vi "FFT_DAS_GUI.vi"() -> ()   [LabVIEW 2018]
doc: "<b>LITVC - ?????????????????????</b>\n\nMeasures, graphs and logs the data from the LITVC cRIO Chassis. Samples 12 analog channels of raw at kilohertz speeds, and controls starting of test data runs, with triggered control of the appropriate solenoid valves . \n\nSystem scaling and other constants are loaded from the \"LITVC_CFG.TXT\" text file at startup. (The order of the lines must remain the same. ) The Operator must supply a data file path and name at startup. This defaults on the cRIO Controller to: \"C:\\Data\". The software then starts data acquisition and logging, as indicated by the blinking green \"Active\" LED.\n\nPressing \"CAL\" after start will calibrate the system to the cross section of the wire rope.\nTo stop the acquisition, press the Stop button in the upper right. This allows the operator to look at the graphs, error indicators, etc on the status tab.\nTo Exit, press the EXIT button on the Status tab.\n\nVersion 1.0.0:\n 1. Initial version\n\n2010_09_30 Michael Ashe\nmichael.ashe@aztera.com\nmichael.ashe@imaginatics.net\n(860) 961-0876 (Cell)"
uses:
  Common/Controls/GUI_Buttons_23x22_W2K.llb/MacroPlay.ctl
  Common/Controls/GUI_Buttons_23x22_W2K.llb/MacroPause.ctl
  Common/Controls/GUI_Buttons_23x22_W2K.llb/MacroStop.ctl
  Common/Controls/BlockStart Button.ctl
  Common/Controls/BlockEnd Button.ctl
  Common/Controls/FFT_DAS Shift Variables.ctl
  Common/COMM_Queues/Command Queue Cluster.ctl
  Common/WRIS_Config Vars Cluster.ctl
  Common/GUI/Enable Controls API.llb/Action.ctl
  Common/Timing/Controls/StateMachineStates_TEST_TDEF.ctl
  Common/COMM_Queues/Command_Queue_Select.ctl
  Common/StateFile.llb/Actions.ctl
  <vilib>/DAQmx/read.llb/DAQmx Read (Analog 1D DBL NChan 1Samp).vi
  <vilib>/DAQmx/write.llb/DAQmx Write (Analog 1D DBL NChan 1Samp).vi
  <vilib>/DAQmx/read.llb/DAQmx Read (Analog 1D Wfm NChan NSamp).vi
  <vilib>/DAQmx/read.llb/DAQmx Read (Counter DBL 1Chan 1Samp).vi
  Common/Globals/FFT_DAS-Editing Variables_GBL.vi
  <vilib>/DAQmx/miscellaneous.llb/DAQmx Fill In Error Info.vi
  <vilib>/measure/madcrms.llb/Basic Averaged DC-RMS for N Chan.vi
  <vilib>/DAQmx/configure/timing.llb/DAQmx Timing (Sample Clock).vi
  <vilib>/DAQmx/create/channels.llb/DAQmx Create Channel (CI-Frequency).vi
  <vilib>/DAQmx/configure/timing.llb/DAQmx Timing (Implicit).vi
  Common/GUI/Enable Controls.lvlib
  <vilib>/measure/NI_MAPro.lvlib
panel:
  out "SaveAbortedTest":bool
  out "Test Data":dbl[](array[numeric])
  out "Flow":i32
  out "GPM":dbl[](array[numeric])
  out "Hz":dbl[](array[numeric])
  out "DAQWrite":errorcluster
  out "Numeric":i32
  out "StopAllLoops":bool
  out "Flow Meter":bool
  out "Thermocouple":bool
  out "DAQ":bool
  in  "Tab Control":T1(tab)
  out "In Range":bool=TRUE
  in  "Go to Previous Step":bool
  out "Supply Pressure":dbl(knob) scale=0.0..400.0 scale format="%#.1f"
  out "Hz":dbl format="%.1f"
  out "Fuel Temp":dbl(slide) scale=0.0..150.0 scale format="%#.1f"
  out "Flow(GPM)":dbl(knob) scale=0.0..2.0 scale format="%#.1f"
  out "Flow(lbs/hr)":dbl(knob) scale=0.0..1000.0 scale format="%#.1f"
  out "Bypass Pressure (psig)":dbl(knob) scale=0.0..50.0 scale format="%#.1f"
  out "Back Pressure":dbl(knob) scale=0.0..300.0 scale format="%#.1f"
  out "Diff. Pressure":dbl(knob) scale=0.0..60.0 scale format="%#.1f"
  in  "Go to Next Step":bool
  in  "BP Reg Manual":bool
  in  "Control Devices":cluster{"BP Regulator":dbl} {"BP Regulator" scale=0.0..100.0 scale format="%#3.2f%"}
  out "Test Status":T2(ring)
  in  "BlkMrkGrp":cluster{"Block Start":T3, "Block End":T4}
  in  "MacroGroup":T8
  in  "Test Table":string[][](table)=[["", "20", "10", "109 ", "200", " ", " ", " ", " ", " ", " ", " ", " ", " ", " "], ["", "40", "22", "160", "200", "", " ", " ", " ", " ", " ", " ", " ", " ", " "], ["", "10", "32", "400", "500", "", " ", " ", " ", " ", " ", " ", " ", " ", " "]] caption="A/M    Current      Dwell            Min Flow       Max Flow       Actual Flow      Hysteresis"
  out "EditLine":i32=65534
  out "EditCol":i32=65534
  in  "StartTest":bool
  in  "StopTest":bool
  out "ATS Number":string
  out "CalDate":string
  in  "PSID Setpoint":dbl
  in  "Pressure Tolerance":dbl
  out "mA Tolerance":dbl
  out "Parameter Table Out 2":string[][](table) caption="Parameter Table + Comment Out"
  out "BP Output":dbl format="%.2g"
  out "Report Path":path
  out "Template Path":path
  out "Version":string
  in  "Send to Excel":bool
  out "Test Table2":string[][](table)=[["", "20", "10", "109 ", "200", " ", " ", " ", " ", " ", " ", " ", " ", " ", " "], ["", "40", "22", "160", "200", "", " ", " ", " ", " ", " ", " ", " ", " ", " "], ["", "10", "32", "400", "500", "", " ", " ", " ", " ", " ", " ", " ", " ", " "]] caption="Table"
  out "Parameter Table Out":string[][](table)
  out "Flow-Current XY Graph":cluster{cluster{"X":dbl, "Y":dbl}[]}[](graph)
  out "Flow Freq":errorcluster
  out "DAQRead":errorcluster
  out "USB TC 01":errorcluster
  out "TM Config File":path
  out "AI Task":refnum<k21>="AI"
  out "FEM Device":tag="Dev1/ctr0"
  out "Report Path":path
  out "TempCorrection":dbl
  out "Flow Cal":dbl[][](array[numeric])
  out "@Temp Cal Fluid":dbl format="%.1g °F"
  out "SG Cal Fluid":dbl format="%#.6g"
  out "SG Cal Corrected":dbl format="%.3g"
  out "Cal Temp Coe":dbl format="%#.6g"
  out "Current Cal Temp":dbl format="%.1g °F"
  out "Flow lbs/hr":dbl format="%.3g"
  out "Flow(GPM)":dbl format="%#.3g"
  out "SG CAL Corrected":dbl format="%#.3g"
  out "Std H20 Mass @60F":dbl format="%#.3g"
  # "SG CAL Corrected ="
  # "Hz"
  # "GPM"
  # "SG Cal Fluid + Cal Temp Coe*(Temp Cal Fluid-Current Fuel Temp)"
  # "Flow (PPH) ="
  # "Flow(gpm)*60*SG CAL Correct *Standard H20 Mass @60F"
  # "\"Flow Calibration.txt\" is located in the application directory.\n\nMake Changes to that file and relaunch the application\nto initialize the new calibration. \n\n\nIf the file does not exist create one with the exact file\nname above.  Add as many points as needed. Example:\n\nHz, GPM\n0, 0\n2, 100\n10, 1010"
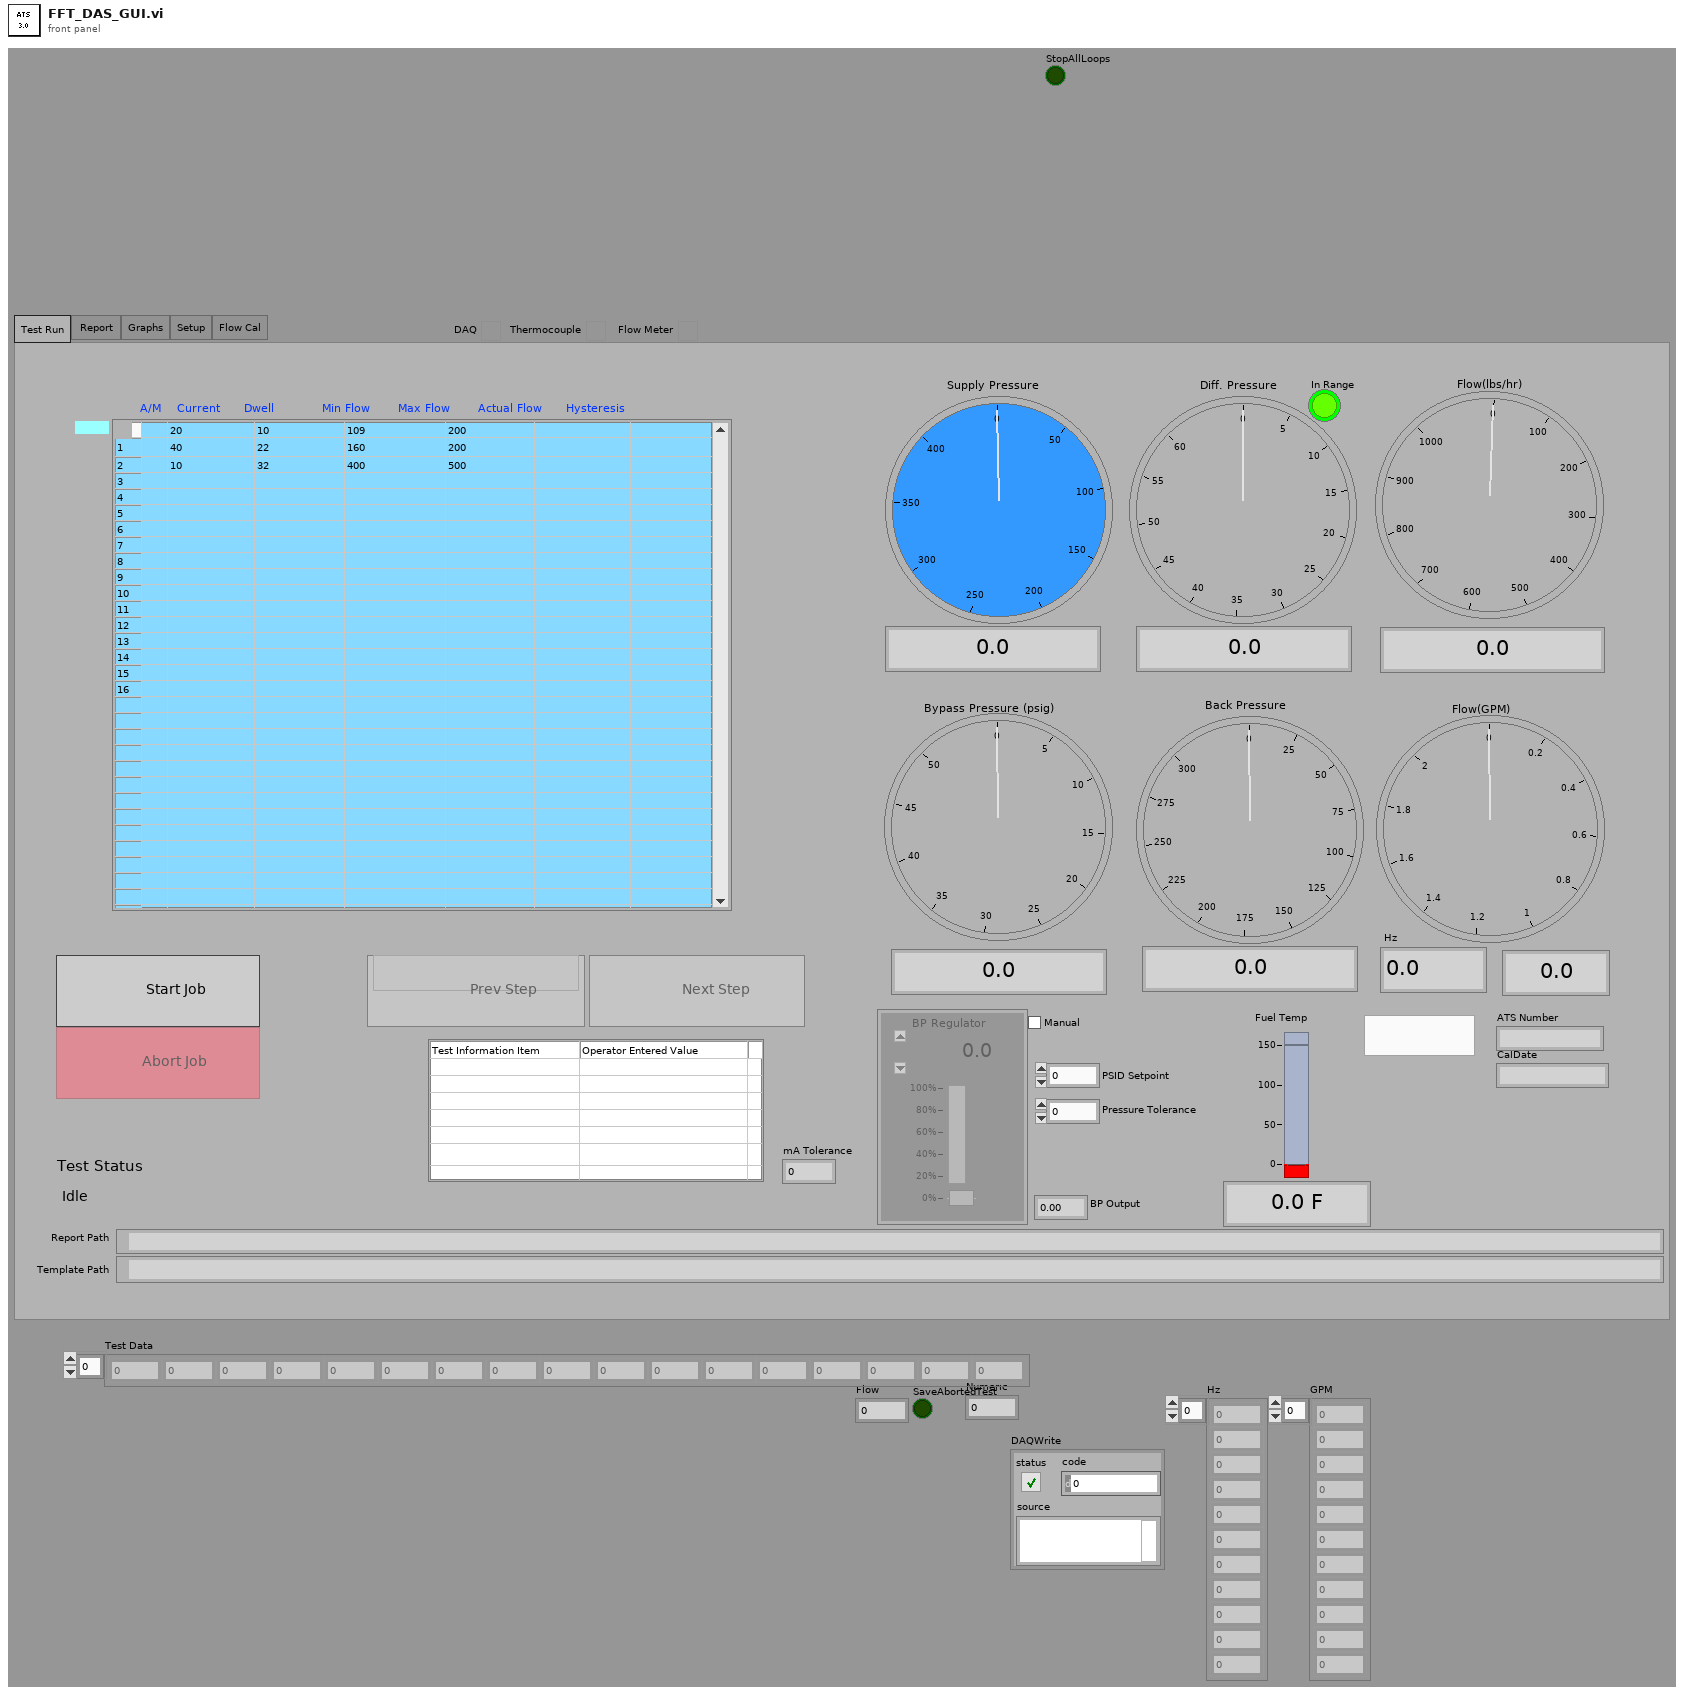
[diagram p1: front panel]
types:
  T1 = enum32{"Test Run", "Report ", "Graphs", "Setup", "Flow Cal"}
  T2 = enum16{"Idle", "Test Running", "Test Paused", "Test Completed"}
  T3 = typedef "BlockStart Button.ctl" = bool
  T4 = typedef "BlockEnd Button.ctl" = bool
  T5 = typedef "MacroPlay.ctl" = bool
  T6 = typedef "MacroPause.ctl" = bool
  T7 = typedef "MacroStop.ctl" = bool
  T8 = cluster{"MacroPlay":T5, "MacroPause":T6, "MacroStop":T7, "MacroName":u16}
  T9 = typedef "FFT_DAS Shift Variables.ctl" = cluster{"queue data":T10, "error":errorcluster, "Q_TO":i32, "WDT_TO":dbl, "LogErrors?":bool, "Main.ini Ref":refnum<k1>, "Connected? 1":bool, "Address 1":string, "Link_Name":string, "Config Vars":T11, "Calibrate":bool, "Cal_Slope-Offset":dbl[][], "TestTable":string[][], "Test Status":enum16{"Idle", "Test Running", "Test Paused", "Test Completed"}, "Parameter Table Out":string[][], "Test Start Time":string, "Test Stop Time":string, "Report Directory":path}
  T10 = typedef "Command Queue Cluster.ctl" = cluster{"Command":string, "Variant Data":variant}
  T11 = typedef "WRIS_Config Vars Cluster.ctl" = cluster{"Distance/Count":dbl, "samples/ch":i32, "Task_TO":dbl, "Kc":dbl, "B":dbl}
  T12 = typedef "Enable Controls.lvlib/Action.ctl" = enum16{"Editor Init", "Init", "Operator Init", "Timed Test Start", "Manual Test Start", "Stop Test", "Close", "Set States"}
  T13 = enum16{"get data", "set data", "Add Data Pair", "initialize"}
  T14 = typedef "StateMachineStates_TEST_TDEF.ctl" = enum16{"Initialize", "Start", "Run Position", "Pause", "Resume", "Get Step", "Force Previous Step", "Force Next Step", "Stay on Current Step"}
  T15 = typedef "Command_Queue_Select.ctl" = enum16{"<no op>", "Destroy Queues", "Send -> State_Machine", "Send -> Client_IO", "Send -> Logging", "Send -> Instrument_IO", "Send -> Tag_Manager", "Send -> Alarms_Shutdowns", "Send -> Control_Loops", "Send -> Server_IO", "Send -> GUI"}
  T16 = typedef "Actions.ctl" = enum16{"Initialize", "Save VI State", "Load VI State", "Delete State", "Get All VI State Names", "Clear All States", "Close Global State File", "Open State File", "Create State File", "Write Data to File", "Exit"}
  T17 = enum8{"Enabled", "Disabled", "Disabled and Grayed Out"}
  T18 = typedef "LVRowAndColumnTypeDef.ctl" = cluster{"Row":i32, "Column":i32}
  T19 = enum16{"STARTUP", "ERROR", "OPEN", "CLOSE", "ENABLE", "DISABLE", "SHUTDOWN"}
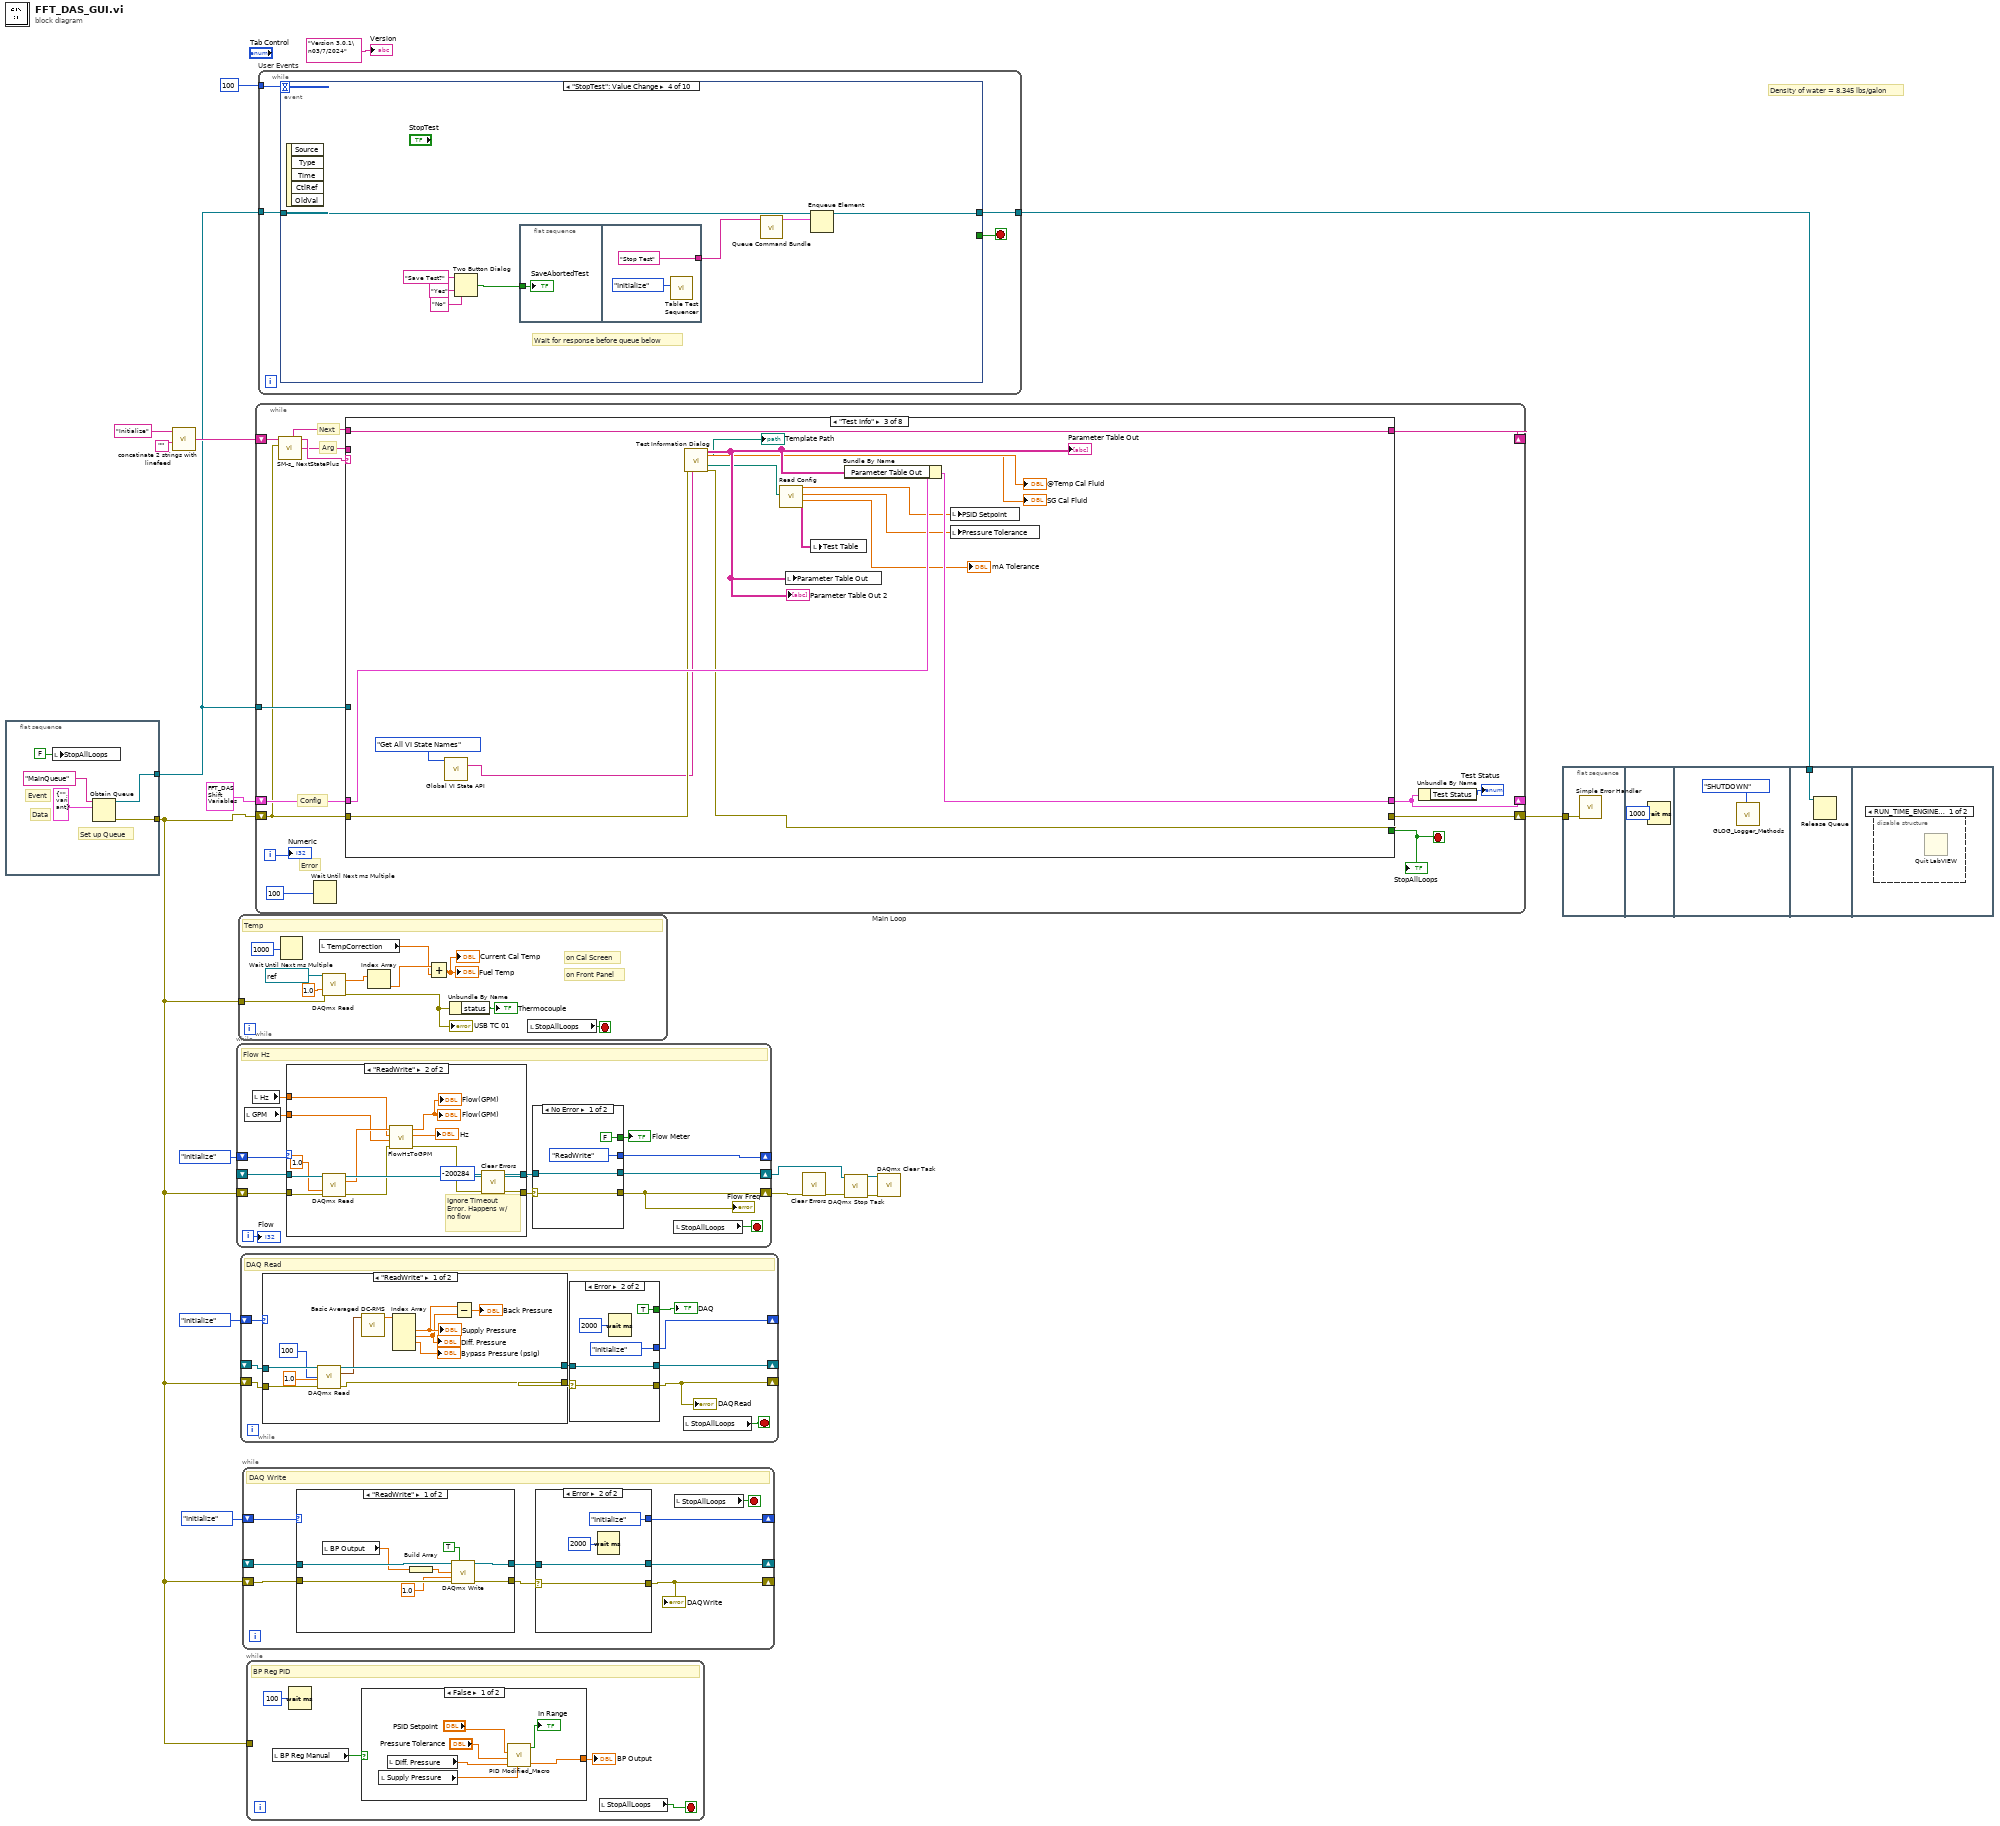
[diagram p0: block diagram]
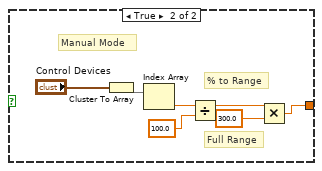
[diagram p2: hidden frame]
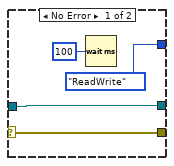
[diagram p3: hidden frame]
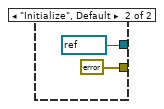
[diagram p4: hidden frame]
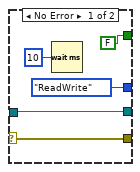
[diagram p5: hidden frame]
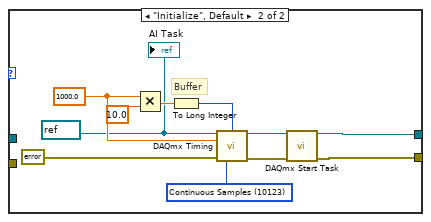
[diagram p6: hidden frame]
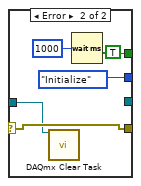
[diagram p7: hidden frame]
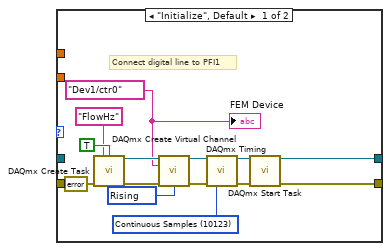
[diagram p8: hidden frame]
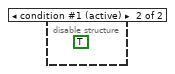
[diagram p9: hidden frame]
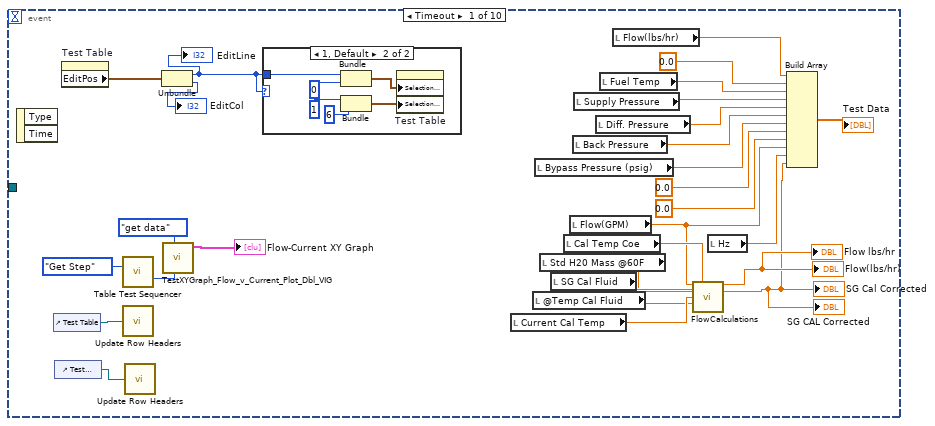
[diagram p10: hidden frame]
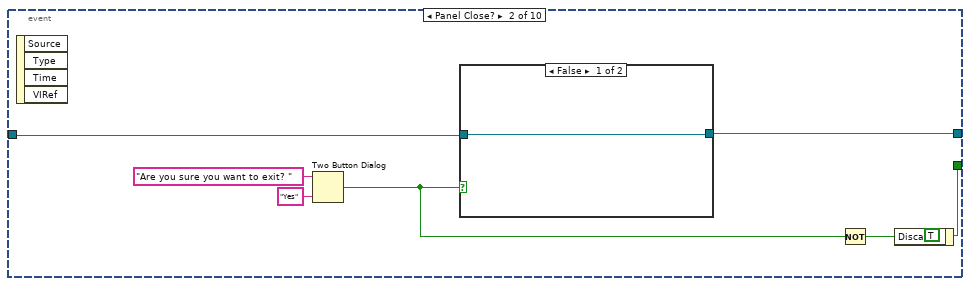
[diagram p12: hidden frame]
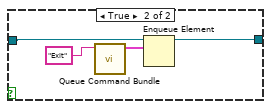
[diagram p13: hidden frame]
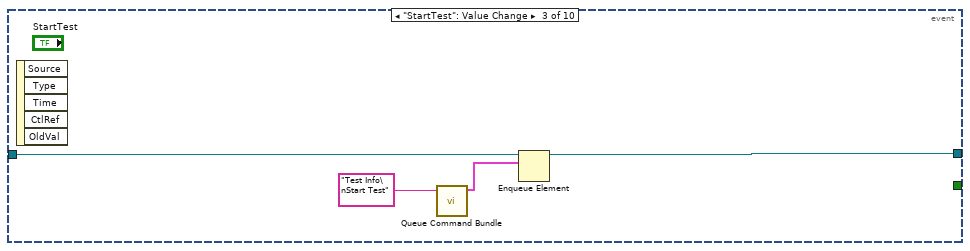
[diagram p14: hidden frame]
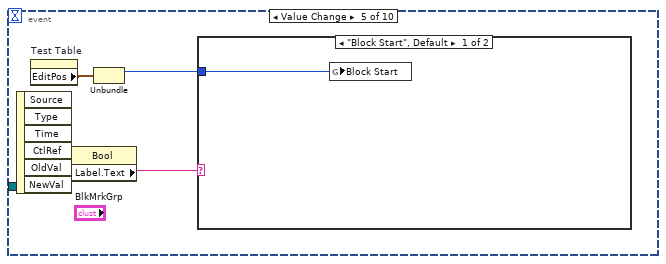
[diagram p15: hidden frame]
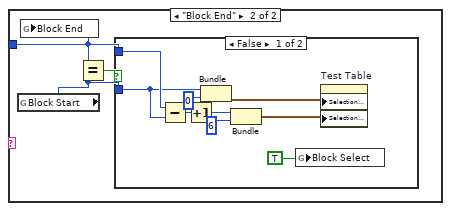
[diagram p16: hidden frame]
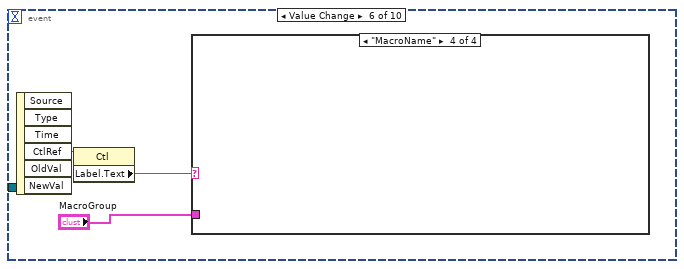
[diagram p18: hidden frame]
diagram:
  # "Density of water = 8.345 lbs/galon"
  n1 = flat-sequence {
    tunnel: [w21] -> w1
    tunnel: [w20] -> w11
    frame #0 {
      # "Data"
      # "Event"
      # "Set up Queue"
      n2 = local write "StopAllLoops"(FALSE ("StopAllLoops")) -> ()
      n3 = Obtain Queue(name (unnamed)="MainQueue", element data type=T10 {"Command"="", "Variant Data"=variant} ("queue data")) -> (queue out=w20:refnum<queue>, error out=w21:errorcluster)  [unwired: 3 in, 1 out]
    }
  }
  n4 = call "concatinate 2 strings with linefeed.vi"("String 2"="", "String 1"="Initialize") -> ("Concatinated OUT"=w18:string)  [unwired: 6 in]
  n5 = while "Flow Hz" {
    shift-right: [w30] -> w6
    shift-left: _ -> [w36]
    shift-right: [w27] -> w9
    shift-left: w1 -> [w35]
    shift-right: [w29] -> _
    shift-left: enum16{"Initialize", "ReadWrite"}."Initialize" -> [w34]
    i -> [w24]
    stop <- w33 stop-if-true
    # "Flow Hz"
    n6 = local read "GPM"() -> (w25:dbl[])
    n7 = local read "Hz"() -> (w26:dbl[])
    n8 = case shown="\"ReadWrite\"" w34 {
      tunnel: [w50 w67] -> w32
      tunnel: w36 -> [_ w72]
      tunnel: [w49 w61] -> w31
      tunnel: w35 -> [_ w71]
      tunnel: w26 -> [_ w65]
      tunnel: w25 -> [_ w64]
      frame "Initialize", Default {
        w47 = 10280 items=["Rising"=10280, "Falling"=10171] ("starting edge")
        w52 = 10123 items=["Finite Samples"=10178, "Continuous Samples"=10123, "Hardware Timed Single Point"=12522] ("sample mode")
        w56 = tag "Dev1/ctr0" ("counter")
        # "Connect digital line to PFI1"
        n9 = call <vilib>:"DAQmx Create Task.vi"("new task name"="FlowHz", "auto cleanup"=TRUE, "error in"=errorcluster {"status"=FALSE, "code"=0, "source"=""}) -> ("task out"=w59:refnum<k21>, "error out"=w55:errorcluster)  [unwired: 11 in]
        n10 = call-poly <vilib>:"DAQmx Create Virtual Channel.vi"("task in"=w59, "counter"=w56, "error in"=w55, "starting edge"=w47) -> ("task out"=w53:refnum<k21>, "error out"=w54:errorcluster)  [unwired: 10 in]
        n11 = call-poly <vilib>:"DAQmx Timing.vi"("task/channels in"=w53, "sample mode"=w52, "error in"=w54) -> ("task out"=w51:refnum<k21>, "error out"=w48:errorcluster)  [unwired: 11 in]
        n12 = call <vilib>:"DAQmx Start Task.vi"("task/channels in"=w51, "error in"=w48) -> ("task out"=w50:refnum<k21>, "error out"=w49:errorcluster)  [unwired: 12 in]
        "FEM Device" <- w56
      }
      frame "ReadWrite" {
        # "Ignore Timeout\nError. Happens w/\nno flow"
        n13 = call-poly <vilib>:"DAQmx Read.vi"("task/channels in"=w72, "timeout"=1.0, "error in"=w71) -> ("task out"=w67:refnum<k21>, "data"=w66:dbl, "error out"=w63:errorcluster)  [unwired: 10 in]
        n14 = call "FlowHzToGPM.vi"("error in"=w63, "GPM"=w64, "Hz"=w65, "Freq"=w66) -> ("error out"=w62:errorcluster, "Flow Hz"=→"Hz":dbl, "FlowGPH"=→"Flow(GPM)" →"Flow(GPM)":dbl)  [unwired: 5 in]
        n15 = call <vilib>:"Clear Errors.vi"("error in (no error)"=w62, "specific error code to clear (0: all)"=-200284) -> ("error out"=w61:errorcluster)  [unwired: 4 in, 1 out]
      }
    }
    n16 = case shown="No Error" w31 {
      selector: w31 -> [w39 w42]
      tunnel: w32 -> [w40 w41]
      tunnel: [w40 _] -> w30
      tunnel: [w39 w42] -> w27
      tunnel: [enum16{"Initialize", "ReadWrite"}."ReadWrite" enum16{"Initialize", "ReadWrite"}."Initialize"] -> w29
      tunnel: [FALSE TRUE] -> w28
      frame No Error {
      }
      frame Error {
        n17 = call <vilib>:"DAQmx Clear Task.vi"("task in"=w41) -> ()  [unwired: 14 in, 1 out]
        n18 = Wait (ms)(milliseconds to wait=u32 1000) -> ()  [unwired: 1 out]
      }
    }
    "Flow Meter" <- w28
    "Flow Freq" <- w27
    n19 = local read "StopAllLoops"() -> (w33:bool)
    "Flow" <- w24
  }
  n20 = while "Temp" {
    tunnel: w1 -> [w77]
    stop <- w83 stop-if-true
    # "on Front Panel"
    # "on Cal Screen"
    # "Temp"
    n21 = Wait Until Next ms Multiple(millisecond multiple=u32 1000) -> ()  [unwired: 1 out]
    n22 = local read "TempCorrection"() -> (w74:dbl)
    n23 = call-poly <vilib>:"DAQmx Read.vi"("task/channels in"=refnum<k21> "Temp", "timeout"=1.0, "error in"=w77) -> ("data"=w81:dbl[], "error out"=w76:errorcluster)  [unwired: 10 in, 1 out]
    "USB TC 01" <- w76
    n24 = Index Array(array=w81) -> (element=w75:dbl)  [unwired: 1 in]
    n25 = Add(x=w75, y=w74) -> (x+y=→"Fuel Temp" →"Current Cal Temp":dbl)
    n26 = Unbundle By Name(w76) -> ("status"=→"Thermocouple":bool)
    n27 = local read "StopAllLoops"() -> (w83:bool)
  }
  n28 = while {
    shift-right: [w87] -> _
    shift-left: enum16{"Initialize", "ReadWrite"}."Initialize" -> [w93]
    shift-right: [w85] -> _
    shift-left: w1 -> [w91]
    shift-right: [w88] -> _
    shift-left: _ -> [w92]
    stop <- w84 stop-if-true
    # "DAQ Read"
    n29 = case shown="\"ReadWrite\"" w93 {
      tunnel: [w113 w118] -> w89
      tunnel: [w112 w116] -> w90
      tunnel: w92 -> [w115 _]
      tunnel: w91 -> [w114 _]
      frame "ReadWrite" {
        n30 = call-poly <vilib>:"DAQmx Read.vi"("task/channels in"=w115, "number of samples per channel"=100, "timeout"=1.0, "error in"=w114) -> ("task out"=w112:refnum<k21>, "data"=w111:waveform(dbl)[], "error out"=w113:errorcluster)  [unwired: 9 in]
        n31 = call-poly <vilib>:"Basic Averaged DC-RMS.vi"("signals in"=w111) -> ("DC values"=w108:dbl[])  [unwired: 7 in, 3 out]
        n32 = Index Array(array=w108) -> (element #1=w107:dbl, element #2=w104:dbl, element #3=→"Bypass Pressure (psig)":dbl)  [unwired: 4 in, 1 out]
        "Supply Pressure" <- w107
        "Diff. Pressure" <- w104
        n33 = Subtract(x=w107, y=w104) -> (x-y=→"Back Pressure":dbl)
      }
      frame "Initialize", Default {
        w120 = 1000.0 ("rate")
        w121 = 10123 items=["Finite Samples"=10178, "Continuous Samples"=10123] ("sample mode")
        w119 = refnum<k21> "AI" ("task out")
        # "Buffer"
        n34 = Multiply(x=w120, y=10.0) -> (x*y=w123:dbl)
        n35 = To Long Integer(number=w123) -> (32bit integer=w122:i32)
        n36 = call-poly <vilib>:"DAQmx Timing.vi"("task/channels in"=w119, "sample mode"=w121, "samples per channel"=w122, "rate"=w120, "error in"=errorcluster {"status"=FALSE, "code"=0, "source"=""}) -> ("task out"=w125:refnum<k21>, "error out"=w126:errorcluster)  [unwired: 9 in]
        n37 = call <vilib>:"DAQmx Start Task.vi"("task/channels in"=w125, "error in"=w126) -> ("task out"=w116:refnum<k21>, "error out"=w118:errorcluster)  [unwired: 12 in]
        "AI Task" <- w119
      }
    }
    n38 = case shown="Error" w89 {
      selector: w89 -> [w97 w102]
      tunnel: w90 -> [w98 w100]
      tunnel: [w98 w100] -> w88
      tunnel: [w97 w102] -> w85
      tunnel: [enum16{"Initialize", "ReadWrite"}."ReadWrite" enum16{"Initialize", "ReadWrite"}."Initialize"] -> w87
      tunnel: [FALSE TRUE] -> w86
      frame No Error {
        n39 = Wait (ms)(milliseconds to wait=u32 10) -> ()  [unwired: 1 out]
      }
      frame Error {
        n40 = Wait (ms)(milliseconds to wait=u32 2000) -> ()  [unwired: 1 out]
      }
    }
    "DAQ" <- w86
    "DAQRead" <- w85
    n41 = local read "StopAllLoops"() -> (w84:bool)
  }
  n42 = while {
    shift-right: [w129] -> _
    shift-left: enum16{"Initialize", "ReadWrite"}."Initialize" -> [w135]
    shift-right: [w128] -> _
    shift-left: w1 -> [w133]
    shift-right: [w130] -> _
    shift-left: _ -> [w134]
    stop <- w127 stop-if-true
    # "DAQ Write"
    n43 = case shown="\"ReadWrite\"" w135 {
      tunnel: [w149 errorcluster {"status"=FALSE, "code"=0, "source"=""} ("error in")] -> w131
      tunnel: [w150 refnum<k21> "AO" ("task out")] -> w132
      tunnel: w134 -> [w151 _]
      tunnel: w133 -> [w148 _]
      frame "ReadWrite" {
        n44 = local read "BP Output"() -> (w145:dbl)
        n45 = Build Array(w145) -> (w144:dbl[])
        n46 = call-poly <vilib>:"DAQmx Write.vi"("task/channels in"=w151, "auto start"=TRUE, "data"=w144, "timeout"=1.0, "error in"=w148) -> ("task out"=w150:refnum<k21>, "error out"=w149:errorcluster)  [unwired: 8 in, 1 out]
      }
      frame "Initialize", Default {
      }
    }
    n47 = case shown="Error" w131 {
      selector: w131 -> [w138 w142]
      tunnel: w132 -> [w139 w141]
      tunnel: [w139 w141] -> w130
      tunnel: [w138 w142] -> w128
      tunnel: [enum16{"Initialize", "ReadWrite"}."ReadWrite" enum16{"Initialize", "ReadWrite"}."Initialize"] -> w129
      frame No Error {
        n48 = Wait (ms)(milliseconds to wait=u32 100) -> ()  [unwired: 1 out]
      }
      frame Error {
        n49 = Wait (ms)(milliseconds to wait=u32 2000) -> ()  [unwired: 1 out]
      }
    }
    "DAQWrite" <- w128
    n50 = local read "StopAllLoops"() -> (w127:bool)
  }
  n51 = while {
    tunnel: w1 -> [_]
    stop <- w154 stop-if-true
    # "BP Reg PID"
    n52 = local read "BP Reg Manual"() -> (w155:bool)
    n53 = Wait (ms)(milliseconds to wait=u32 100) -> ()  [unwired: 1 out]
    n54 = case shown="False" w155 {
      tunnel: [w160 w166] -> w157
      frame False {
        n55 = local read "Supply Pressure"() -> (w161:dbl)
        n56 = local read "Diff. Pressure"() -> (w162:dbl)
        n57 = call "PID Modified_Macro.vi"("Diff Press Setpoint"="PSID Setpoint", "Supply Pressure"=w161, "Tolerance"="Pressure Tolerance", "Differential Pressure"=w162) -> ("In Range?"=→"In Range":bool, "BP Output"=w160:dbl)  [unwired: 5 in]
      }
      frame True {
        # "% to Range"
        # "Full Range"
        # "Manual Mode"
        n58 = Cluster To Array(cluster="Control Devices") -> (array=w170:dbl[])
        n59 = Index Array(array=w170) -> (element=w168:dbl)  [unwired: 1 in]
        n60 = Divide(x=w168, y=100.0) -> (x/y=w165:dbl)
        n61 = Multiply(x=w165, y=300.0) -> (x*y=w166:dbl)
      }
    }
    "BP Output" <- w157
    n62 = local read "StopAllLoops"() -> (w154:bool)
  }
  n63 = while "Main Loop" {
    shift-right: [w183] -> _
    shift-left: w18 -> [w175]
    shift-right: [w174] -> _
    shift-left: T9 {"queue data"={"Command"="", "Variant Data"=variant}, "error"={"status"=FALSE, "code"=0, "source"=""}, "Q_TO"=0, "WDT_TO"=0.0, "LogErrors?"=FALSE, "Main.ini Ref"=refnum, "Connected? 1"=FALSE, "Address 1"="", "Link_Name"="", "Config Vars"={"Distance/Count"=0.0, "samples/ch"=0, "Task_TO"=0.0, "Kc"=0.0, "B"=0.0}, "Calibrate"=FALSE, "Cal_Slope-Offset"=[], "TestTable"=[], "Test Status"=enum."Idle", "Parameter Table Out"=[], "Test Start Time"="", "Test Stop Time"="", "Report Directory"=path ""} ("VARS WRIS") -> [w184]
    shift-right: [w172] -> w14
    shift-left: w1 -> [w176]
    tunnel: w11 -> [w177]
    i -> [w171]
    stop <- w178 stop-if-true
    # "Arg"
    # "Next"
    # "Error"
    # "Config"
    n64 = call "SM-s_ NextStatePlus.vi"("error?"=w176, "States String"=w175) -> ("Argument"=w181:string, "Current State"=w182:string, "Next States"=w180:string)  [unwired: 7 in]
    n65 = Wait Until Next ms Multiple(millisecond multiple=u32 100 ("Loop Wait (mSec)")) -> ()  [unwired: 1 out]
    n66 = case shown="\"Test Info\"" w182 {
      tunnel: w184 -> [w201 w216 w306 w312 w337 w350 w378 w403]
      tunnel: [w186 w224 w308 w326 w342 w362 w373 w403] -> w174
      tunnel: w176 -> [w192 w221 w305 w311 w336 w359 w376 w401]
      tunnel: [w191 w217 w302 w311 w336 w359 w376 w401] -> w172
      tunnel: [w202 w219 w309 w323 w339 "Check Queue" ("Next States") w377 w404] -> w183
      tunnel: w181 -> [_ _ _ _ _ _ _ _]
      tunnel: w180 -> [w202 w220 w309 w324 w339 _ w377 w404]
      tunnel: [_ _ _ _ _ _ _ TRUE] -> w178
      tunnel: w177 -> [_ w225 _ _ _ _ _ _]
      frame "Initialize" {
        w189 = 0.5 ("Pressure Tolerance")
        # "Cal Fluid = MIL-PRF-7024"
        n67 = control-ref of="Test Table2"() -> (w208:refnum<vi>)
        n68 = control-ref of="Test Table"() -> (w207:refnum<vi>)
        n69 = call "Table Color Init-Reset.vi"("Test Table"=w208) -> ()  [unwired: 11 in]
        n70 = call "Table Color Init-Reset.vi"("Test Table"=w207) -> ()  [unwired: 11 in]
        n71 = property on="BP Reg Manual" class="Bool (strict)"("Val(Sgnl)"=FALSE ("Value (Signaling)")) -> ()  [unwired: 2 in, 2 out]
        n72 = call "Enable Controls.vi"("Enabled State"=Action."Init") -> ("error out"=w197:errorcluster)  [unwired: 10 in]
        n73 = call "Table Test Sequencer.vi"("Action"=StateMachineStates_TEST_TDEF."Initialize") -> ()  [unwired: 3 in, 8 out]
        n74 = call "Enable Controls.vi"("error in"=w197, "Enabled State"=Action."Editor Init") -> ()  [unwired: 9 in, 1 out]
        n75 = call "TestXYGraph_Flow_v_Current_Plot_Dbl_VIG.vi"("Plot Index/Size"=3, "Point index/size"=0, "Operation"=T13."initialize") -> ()  [unwired: 6 in, 3 out]
        n76 = call "Load Flow Calibration.vi"() -> ("CalDate"=→"CalDate":string, "ATSNumber"=→"ATS Number":string, "GPM Output"=w210:dbl[], "Hz Output"=w209:dbl[])  [unwired: 8 in]
        "Hz" <- w209
        "GPM" <- w210
        n77 = local write "Tab Control"(enum32{"Test Run", "Report ", "Graphs", "Setup"}."Test Run" ("Tab Control")) -> ()
        n78 = Build Array(w209, w210) -> (w211:dbl[][])
        n79 = Transpose 2D Array(2D array=w211) -> (transposed array=→"Flow Cal":dbl[][])
        n80 = local write "Pressure Tolerance"(w189) -> ()
        n81 = local write "mA Tolerance"(w189) -> ()
        n82 = local write "PSID Setpoint"(50.0 ("PSID Setpoint")) -> ()
        n83 = local write "@Temp Cal Fluid"(70.0 ("Ti")) -> ()
        n84 = local write "SG Cal Fluid"(0.77 ("SGi")) -> ()
        n85 = call "Read TM Config.vi"("error in (no error)"=w192) -> ("error out"=w191:errorcluster, "Standard H20 Mass @ 60"=→"Std H20 Mass @60F":dbl, "Cal Temp Coefficient"=→"Cal Temp Coe":dbl, "Config Path ourt"=→"TM Config File":path, "TempCorrection"=→"TempCorrection":dbl, "Report Path"=w185:path)  [unwired: 5 in]
        "Report Path" <- w185
        n86 = Bundle By Name(cluster=w201, "Report Directory"=w185) -> (w186:T9)
      }
      frame "Check Queue", Default {
        # "incoming Cmd"
        n87 = call "Queue Command Read & Parse.vi"("Command_Q"=w225) -> ("Variant Data"=w223:variant, "Command"=w222:string)  [unwired: 7 in, 2 out]
        n88 = case shown="\"Timeout\", Default" w222 {
          selector: w222 -> [w230 _ _]
          tunnel: w216 -> [w227 w247 w256]
          tunnel: [w226 w247 w256] -> w224
          tunnel: w223 -> [_ _ w252]
          tunnel: [w234 "Exit" w259] -> w218
          tunnel: w221 -> [w236 w245 w251]
          tunnel: [w236 w245 w248] -> w217
          frame "Timeout", Default {
            # "Push incomming command\nto top of command stack"
            n89 = Unbundle By Name(w227) -> ("Test Status"=w235:T2)
            n90 = Equal?(x=w230, y="Timeout") -> (x = y?=w231:bool)
            n91 = case shown="\"Test Completed\"" w235 {
              tunnel: ["" ("element") "Run Test" ("element") "Stop Test\nSend to Excel" ("element")] -> w233
              tunnel: w227 -> [w237 w239 w243]
              tunnel: [w237 w239 w242] -> w226
              frame "Idle", Default {
              }
              frame "Test Running" {
              }
              frame "Test Completed" {
                n92 = Bundle By Name(cluster=w243, "Test Status"=T2."Idle") -> (w242:T9)
              }
            }
            n93 = Select(t="", s=w231, f=w230) -> (s? t:f=w229:string)
            n94 = call "concatinate 2 strings with linefeed.vi"("String 2"=w233, "String 1"=w229) -> ("Concatinated OUT"=w234:string)  [unwired: 6 in]
          }
          frame "Exit" {
          }
          frame "ReceiveCMD" {
            # "This will be filled in with commands to\nStartTest:FileNamePath\nStopTest\nCalibrate"
            n95 = Variant To Data(error in=w251, type="", Variant=w252) -> (data=w255:string, error out=w253:errorcluster)
            n96 = Unflatten From String(type=T10 {"Command"="", "Variant Data"=variant} ("queue data"), binary string=w255, error in (no error)=w253) -> (value=w249:T10, error out=w248:errorcluster)  [unwired: 2 in, 1 out]
            n97 = Unbundle By Name(w249) -> ("Command"=w258:string, "Variant Data"=w257:variant)
            n98 = case shown="\"ListDataFiles\"" w258 {
              selector: w258 -> [_ w261 w266 w269 _ _]
              tunnel: ["Error Handle" ("element") w261 w266 w269 "" ""] -> w259
              tunnel: w257 -> [_ _ w265 _ _ w284]
              frame "", Default {
              }
              frame "Calibrate" {
              }
              frame "Init - Datalog" {
                n99 = Variant To Data(type=path "", Variant=w265) -> (data=w264:path, error out=w263:errorcluster)  [unwired: 1 in]
                n100 = call "WRIS_DataFilePath_VIG.vi"("Operation"=enum16{"get data", "set data"}."set data", "error in"=w263, "DataFilePath_in"=w264) -> ()  [unwired: 7 in, 2 out]
              }
              frame "Stop - Datalogging" {
                n101 = call "WRIS_DataFilePath_VIG.vi"("Operation"=enum16{"get data", "set data"}."set data", "DataFilePath_in"=path "") -> ()  [unwired: 8 in, 2 out]
              }
              frame "ListDataFiles" {
                n102 = call <userlib>:"Current VIs Parent Directory__ogtk.vi"("Relative path (.)"=path "Data files") -> ("Parent Directory (+ Relative)"=w277:path)  [unwired: 4 in]
                n103 = List Folder(path=w277) -> (filenames=w271:string[])  [unwired: 3 in, 3 out]
                n104 = call "Queue Command Bundle.vi"("Variant Data"=w271, "Command"="DataFileList" ("element")) -> ("main window queue datatype"=w273:T10)  [unwired: 9 in]
                n105 = To Variant(anything=w273) -> (Variant=w272:variant)
                n106 = call "API Queue Manager.vi"("Q_Select"=Command_Queue_Select."Send -> Client_IO", "Variant Data"=w272, "Command"="SendSTATUS") -> ()  [unwired: 7 in, 2 out]
              }
              frame "GetDataFile" {
                n107 = Variant To Data(type="", Variant=w284) -> (data=w283:string)  [unwired: 1 in, 1 out]
                n108 = call <userlib>:"Current VIs Parent Directory__ogtk.vi"("Relative path (.)"=path "Data files") -> ("Parent Directory (+ Relative)"=w286:path)  [unwired: 4 in]
                n109 = Build Path(base path=w286, name or relative path=w283) -> (appended path=w282:path)
                n110 = Read from Text File(file (use dialog)=w282, count=-1) -> (text=w281:string)  [unwired: 2 in, 3 out]
                n111 = call "Queue Command Bundle.vi"("Variant Data"=w281, "Command"="DataFile" ("element")) -> ("main window queue datatype"=w289:T10)  [unwired: 9 in]
                n112 = To Variant(anything=w289) -> (Variant=w288:variant)
                n113 = call "API Queue Manager.vi"("Q_Select"=Command_Queue_Select."Send -> Client_IO", "Variant Data"=w288, "Command"="SendSTATUS") -> ()  [unwired: 7 in, 2 out]
              }
            }
          }
        }
        n114 = call "concatinate 2 strings with linefeed.vi"("String 2"=w220, "String 1"=w218) -> ("Concatinated OUT"=w219:string)  [unwired: 6 in]
      }
      frame "Test Info" {
        n115 = call "Global VI State API.vi"("Action"=Actions."Get All VI State Names") -> ("VI States"=w303:string[])  [unwired: 12 in, 2 out]
        n116 = call "Test Information Dialog.vi"("error in"=w305, "Part Numbers"=w303) -> ("Temp  Out"=→"@Temp Cal Fluid":dbl, "Specific Gravity Out"=→"SG Cal Fluid":dbl, "Parameter Table Out"=w307:string[][], "Report Template"=→"Template Path":path, "Config Path"=w301:path, "error out"=w302:errorcluster)  [unwired: 7 in, 1 out]
        "Parameter Table Out" <- w307
        "Parameter Table Out 2" <- w307
        n117 = call "Read Config.vi"("Config Path"=w301) -> ("Test Table"=w300:string[][], "C_Tol"=→"mA Tolerance":dbl, "P_Tol"=w295:dbl, "PSID"=w294:dbl)  [unwired: 6 in, 1 out]
        n118 = local write "Parameter Table Out"(w307) -> ()
        n119 = local write "Test Table"(w300) -> ()
        n120 = Bundle By Name(cluster=w306, "Parameter Table Out"=w307) -> (w308:T9)
        n121 = local write "PSID Setpoint"(w294) -> ()
        n122 = local write "Pressure Tolerance"(w295) -> ()
      }
      frame "Start Test" {
        n123 = control-ref of="Test Table"() -> (w321:refnum<vi>)
        n124 = Array Size(array="Test Table") -> (size(s)=w318:i32[])
        n125 = call "Table Color Init-Reset.vi"("Test Table"=w321) -> ()  [unwired: 11 in]
        n126 = Index Array(array=w318) -> (element=w314:i32)  [unwired: 1 in]
        n127 = control-ref of="Test Table2"() -> (w313:refnum<vi>)
        n128 = call "Table Color Init-Reset.vi"("Test Table"=w313) -> ()  [unwired: 11 in]
        n129 = call "TestXYGraph_Flow_v_Current_Plot_Dbl_VIG.vi"("Plot Index/Size"=3, "Point index/size"=w314, "Operation"=T13."initialize") -> ()  [unwired: 6 in, 3 out]
        n130 = flat-sequence {
          tunnel: "Test Table" -> [w332]
          frame #0 {
            n131 = call "Table Test Sequencer.vi"("Action"=StateMachineStates_TEST_TDEF."Initialize") -> ()  [unwired: 3 in, 8 out]
          }
          frame #1 {
            n132 = local read "Test Table"() -> (w331:string[][])
            n133 = call "Update Table with Sensor Data.vi"("Test Table In"=w331, "Number of Sensors"=12) -> ("Test Table Out"=w330:string[][])  [unwired: 8 in, 5 out]
            n134 = local write "Test Table"(w330) -> ()
            n135 = call "Enable Controls.vi"("Enabled State"=Action."Manual Test Start") -> ()  [unwired: 10 in, 1 out]
          }
          frame #2 {
            n136 = call "Table Test Sequencer.vi"("Action"=StateMachineStates_TEST_TDEF."Start", "Test Table"=w332) -> ()  [unwired: 2 in, 8 out]
          }
          frame #3 {
            n137 = call "Table Test Sequencer.vi"("Action"=StateMachineStates_TEST_TDEF."Pause") -> ()  [unwired: 3 in, 8 out]
          }
        }
        n138 = Get Date/Time String(want seconds? (F)=TRUE) -> (time string=w320:string)  [unwired: 2 in, 1 out]
        n139 = local write "SaveAbortedTest"(TRUE ("SaveAbortedTest")) -> ()
        n140 = Bundle By Name(cluster=w312, "TestTable"="Test Table", "Test Status"=T2."Test Running", "Test Start Time"=w320) -> (w326:T9)
        n141 = call "concatinate 2 strings with linefeed.vi"("String 2"="Run Test" ("element"), "String 1"=w324) -> ("Concatinated OUT"=w323:string)  [unwired: 6 in]
      }
      frame "Stop Test" {
        n142 = flat-sequence {
          frame #0 {
            n143 = control-ref of="Test Table"() -> (w345:refnum<vi>)
            n144 = control-ref of="Test Table2"() -> (w344:refnum<vi>)
            n145 = call "Table Test Sequencer.vi"("Action"=StateMachineStates_TEST_TDEF."Get Step") -> ("Current Step ID"=w343:i32)  [unwired: 3 in, 7 out]
            n146 = call "Table Color Clear Select.vi"("Current Step ID"=w343, "Test Table"=w345) -> ()  [unwired: 10 in]
            n147 = call "Table Color Clear Select.vi"("Current Step ID"=w343, "Test Table"=w344) -> ()  [unwired: 10 in]
          }
          frame #1 {
            n148 = control-ref of="Test Table"() -> (w347:refnum<vi>)
            n149 = call "Table Color Init-Reset.vi"("Test Table"=w347) -> ()  [unwired: 11 in]
          }
        }
        n150 = call "Enable Controls.vi"("Enabled State"=Action."Editor Init") -> ()  [unwired: 10 in, 1 out]
        n151 = Get Date/Time String(want seconds? (F)=TRUE) -> (time string=w340:string)  [unwired: 2 in, 1 out]
        n152 = Bundle By Name(cluster=w337, "Test Status"=T2."Test Completed", "Test Stop Time"=w340) -> (w342:T9)
      }
      frame "Run Test" {
        n153 = Unbundle By Name(w350) -> ("Test Status"=w353:T2)
        n154 = local read "Test Table"() -> (w357:string[][])
        n155 = control-ref of="Test Table"() -> (w358:refnum<vi>)
        n156 = call "Table Test Sequencer.vi"("Action"=StateMachineStates_TEST_TDEF."Run Position") -> ("Test Running"=w354:bool, "Current Step ID"=w351:i32)  [unwired: 3 in, 6 out]
        n157 = case shown="\"Test Running\"" w353 {
          selector: w353 -> [w364 _]
          tunnel: w354 -> [_ w366]
          tunnel: [w364 w365] -> w352
          frame "Idle", Default {
          }
          frame "Test Running" {
            n158 = Select(t=T2."Test Running" ("Test Status"), s=w366, f=T2."Test Completed" ("Test Status")) -> (s? t:f=w365:T2)
          }
        }
        n159 = call "Table Color Update.vi"("Value"=w357, "Current Step ID"=w351, "Test Table"=w358) -> ()  [unwired: 9 in]
        n160 = local read "Test Data"() -> (w348:dbl[])
        n161 = Bundle By Name(cluster=w350, "queue data.Variant Data"=variant, "Calibrate"=FALSE, "Test Status"=w352) -> (w362:T9)
        n162 = call "Update Table with Sensor Data.vi"("Test Table In"=w357, "Test Data"=w348, "Number of Sensors"=12) -> ("Test Table Out"=w356:string[][])  [unwired: 7 in, 5 out]
        "Test Table2" <- w356
        n163 = local write "Test Table"(w356) -> ()
        n164 = flat-sequence {
          tunnel: w351 -> [w370]
          tunnel: w356 -> [w369]
          frame #0 {
            n165 = control-ref of="Test Table2"() -> (w371:refnum<vi>)
            n166 = call "Table Color Update.vi"("Value"=w369, "Current Step ID"=w370, "Test Table"=w371) -> ()  [unwired: 9 in]
          }
        }
      }
      frame "Send to Excel" {
        n167 = local read "SaveAbortedTest"() -> (w375:bool)
        n168 = case shown="True" w375 {
          tunnel: w378 -> [_ w394]
          tunnel: [path "" w380] -> w372
          frame False {
          }
          frame True {
            n169 = Unbundle By Name(w394) -> ("Report Directory"=w385:path, "Parameter Table Out"=w387:string[][], "Test Start Time"=w396:string, "Test Stop Time"=w395:string)
            n170 = call <vilib>:"Check if File or Folder Exists.vi"("path"=w385) -> ("file or folder exists?"=w391:bool, "dup path"=w390:path)  [unwired: 8 in, 1 out]
            n171 = local read "Template Path"() -> (w383:path)
            n172 = case shown="False" w391 {
              tunnel: w390 -> [w398 w400]
              tunnel: [w399 w400] -> w384
              frame False {
                n173 = Create Folder(path (use dialog)=w398) -> (created path=w399:path)  [unwired: 2 in, 2 out]
              }
              frame True {
              }
            }
            n174 = Index Array(array=w387, index (col) #1=0 ("disabled index (col)"), index (col) #2=1 ("index (col)")) -> (element #2=w386:string[])  [unwired: 2 in, 1 out]
            n175 = call "Format Test Filename.vi"("Parameter Table In"=w386, "start path"=w384) -> ("Full Path"=w382:path)
            n176 = Copy(9:TRUE ("overwrite (F)"), 10:w382, 11:w383) -> (3:w380:path)  [unwired: 2 in, 2 out]
            n177 = local read "Test Table"() -> (w397:string[][])
            n178 = local read "ATS Number"() -> (w393:string)
            n179 = local read "CalDate"() -> (w392:string)
            n180 = call "Generate ATS Excel Report.vi"("Test Info"=w387, "Test_End_Time"=w395, "ATS Number"=w393, "Test_Start_Time"=w396, "Test Table"=w397, "Cal Date"=w392, "template"=w380) -> ()  [unwired: 8 in, 1 out]
          }
        }
        "Report Path" <- w372
        n181 = Bundle By Name(cluster=w378, "Test Status"=T2."Idle") -> (w373:T9)
      }
      frame "Exit" {
      }
    }
    "StopAllLoops" <- w178
    n182 = Unbundle By Name(w174) -> ("Test Status"=→"Test Status":T2)
    "Numeric" <- w171
  }
  n183 = while "User Events" {
    tunnel: w11 -> [w407]
    tunnel: 100 -> [w406]
    tunnel: [w405] -> w15
    stop <- w408 stop-if-true
    n184 = event shown="[3] \"StopTest\": Value Change" {
      selector: _ -> [_ _ _ _ _ _ _ _ _ _]
      dyn-events: _ -> [_ _ _ _ _ _ _ _ _ _]
      timeout: w406 -> [_ _ _ _ _ _ _ _ _ _]
      tunnel: [_ TRUE ("Exit") _ _ _ _ _ _ _ _] -> w408
      tunnel: w407 -> [_ w449 w458 w466 _ _ _ _ w496 w498]
      tunnel: [_ w448 w455 w464 _ _ _ _ w496 w497] -> w405
      event Timeout {
        n185 = event-data() -> ()  [unwired: 1 in, 2 out]
        n186 = control-ref of="Test Table"() -> (w435:refnum<vi>)
        n187 = control-ref of="Test Table2"() -> (w432:refnum<vi>)
        n188 = property on="Test Table" class="Tbl (strict)"() -> ("EditPos"=w436:T18)  [unwired: 2 in, 2 out]
        n189 = call "Table Test Sequencer.vi"("Action"=StateMachineStates_TEST_TDEF."Get Step") -> ("Current Step ID"=w430:i32)  [unwired: 3 in, 7 out]
        n190 = call "Update Row Headers.vi"("Test Table"=w435) -> ()
        n191 = call "Update Row Headers.vi"("Test Table"=w432) -> ()
        n192 = Unbundle(w436) -> ("Row"=w428:i32, "Column"=→"EditCol":i32)
        "EditLine" <- w428
        n193 = call "TestXYGraph_Flow_v_Current_Plot_Dbl_VIG.vi"("Point index/size"=w430, "Operation"=T13."get data") -> ("XY Graph"=→"Flow-Current XY Graph":cluster{cluster{"X":dbl, "Y":dbl}[]}[])  [unwired: 7 in, 2 out]
        n194 = case shown="1, Default" w428 {
          tunnel: w428 -> [_ w437]
          frame -2 {
          }
          frame 1, Default {
            n195 = Bundle("Row"=w437, 0) -> (w439:cluster{"Row":i32, i32})  [unwired: 1 in]
            n196 = Bundle(1, 6) -> (w438:cluster{i32, i32})  [unwired: 1 in]
            n197 = property on="Test Table" class="Tbl (strict)"("Selection Start"=w439, "Selection Size"=w438) -> ()  [unwired: 2 in, 2 out]
          }
        }
        n198 = local read "Current Cal Temp"() -> (w420:dbl)
        n199 = local read "@Temp Cal Fluid"() -> (w419:dbl)
        n200 = local read "Bypass Pressure (psig)"() -> (w414:dbl)
        n201 = local read "Std H20 Mass @60F"() -> (w417:dbl)
        n202 = local read "SG Cal Fluid"() -> (w418:dbl)
        n203 = local read "Cal Temp Coe"() -> (w416:dbl)
        n204 = local read "Flow(GPM)"() -> (w411:dbl)
        n205 = local read "Back Pressure"() -> (w422:dbl)
        n206 = local read "Supply Pressure"() -> (w424:dbl)
        n207 = local read "Diff. Pressure"() -> (w423:dbl)
        n208 = local read "Fuel Temp"() -> (w425:dbl)
        n209 = local read "Flow(lbs/hr)"() -> (w421:dbl)
        n210 = call "FlowCalculations.vi"("FlowGPH"=w411, "Temp Coe"=w416, "SGH20"=w417, "Fuel Temp"=w420, "SGi"=w418, "Ti"=w419) -> ("Flow Lb/hr"=→"Flow(lbs/hr)" →"Flow lbs/hr":dbl, "SGCal"=w409:dbl)  [unwired: 7 in, 1 out]
        "SG Cal Corrected" <- w409
        "SG CAL Corrected" <- w409
        n211 = local read "Hz"() -> (w410:dbl)
        n212 = Build Array(w421, 0.0 ("element"), w425, w424, w423, w422, w414, 0.0 ("element"), 0.0 ("element"), w411, w410, w409) -> (→"Test Data":dbl[])
      }
      event Panel Close? {
        n213 = event-data() -> ()  [unwired: 1 in, 4 out]
        n214 = Two Button Dialog(message="Are you sure you want to exit? ", 2:"Yes" ("T button name (\"OK\")")) -> (T button?=w444:bool)  [unwired: 1 in]
        n215 = case shown="False" w444 {
          tunnel: w449 -> [w450 w454]
          tunnel: [w450 w451] -> w448
          frame False {
          }
          frame True {
            n216 = call "Queue Command Bundle.vi"("Command"="Exit" ("element")) -> ("main window queue datatype"=w452:T10)  [unwired: 10 in]
            n217 = Enqueue Element(queue=w454, element=w452) -> (queue out=w451:refnum<queue>)  [unwired: 2 in, 2 out]
          }
        }
        n218 = Not(x=w444) -> (.not. x?=w445:bool)
        n219 = event-data("Discard?"=w445) -> ()  [unwired: 1 in, 1 out]
      }
      event "StartTest": Value Change {
        n220 = event-data() -> ()  [unwired: 1 in, 5 out]
        n221 = call "Queue Command Bundle.vi"("Command"="Test Info\nStart Test" ("element")) -> ("main window queue datatype"=w456:T10)  [unwired: 10 in]
        n222 = Enqueue Element(queue=w458, element=w456) -> (queue out=w455:refnum<queue>)  [unwired: 2 in, 2 out]
      }
      event "StopTest": Value Change {
        # "Wait for response before queue below"
        n223 = event-data() -> ()  [unwired: 1 in, 5 out]
        n224 = Two Button Dialog(message="Save Test?", 1:"No" ("F button name (\"Cancel\")"), 2:"Yes" ("T button name (\"OK\")")) -> (T button?=w460:bool)
        n225 = flat-sequence {
          tunnel: w460 -> [w467]
          tunnel: ["Stop Test" ("element")] -> w459
          frame #0 {
            "SaveAbortedTest" <- w467
          }
          frame #1 {
            n226 = call "Table Test Sequencer.vi"("Action"=StateMachineStates_TEST_TDEF."Initialize") -> ()  [unwired: 3 in, 8 out]
          }
        }
        n227 = call "Queue Command Bundle.vi"("Command"=w459) -> ("main window queue datatype"=w465:T10)  [unwired: 10 in]
        n228 = Enqueue Element(queue=w466, element=w465) -> (queue out=w464:refnum<queue>)  [unwired: 2 in, 2 out]
      }
      event Value Change {
        n229 = event-data() -> ("CtlRef"=w473:refnum<vi>)  [unwired: 1 in, 5 out]
        n230 = property on="Test Table" class="Tbl (strict)"() -> ("EditPos"=w471:T18)  [unwired: 2 in, 2 out]
        n231 = property class="Bool"(reference=w473) -> ("Label.Text"=w472:string)  [unwired: 1 in, 2 out]
        n232 = Unbundle(w471) -> ("Row"=w470:i32)  [unwired: 1 out]
        n233 = case shown="\"Block Start\", Default" w472 {
          tunnel: w470 -> [w474 w477]
          frame "Block Start", Default {
            n234 = global write "FFT_DAS-Editing Variables_GBL.vi" "Block Start"(w474) -> ()
          }
          frame "Block End" {
            n235 = global read "FFT_DAS-Editing Variables_GBL.vi" "Block Start"() -> (w476:i32)
            n236 = global write "FFT_DAS-Editing Variables_GBL.vi" "Block End"(w477) -> ()
            n237 = Equal?(x=w477, y=w476) -> (x = y?=w475:bool)
            n238 = case shown="False" w475 {
              tunnel: w477 -> [w481 _]
              tunnel: w476 -> [w480 _]
              frame False {
                n239 = Subtract(x=w481, y=w480) -> (x-y=w484:i32)
                n240 = Increment(x=w484) -> (x+1=w485:i32)
                n241 = Bundle("Block Start"=w480, 0) -> (w479:cluster{"Block Start":i32, i32})  [unwired: 1 in]
                n242 = Bundle(w485, 6) -> (w478:cluster{i32, i32})  [unwired: 1 in]
                n243 = global write "FFT_DAS-Editing Variables_GBL.vi" "Block Select"(TRUE) -> ()
                n244 = property on="Test Table" class="Tbl (strict)"("Selection Start"=w479, "Selection Size"=w478) -> ()  [unwired: 2 in, 2 out]
              }
              frame True {
              }
            }
          }
        }
      }
      event "MacroGroup.MacroName": Value Change {
        n245 = event-data() -> ("CtlRef"=w489:refnum<vi>)  [unwired: 1 in, 5 out]
        n246 = property class="Ctl"(reference=w489) -> ("Label.Text"=w487:string)  [unwired: 1 in, 2 out]
        n247 = case shown="\"MacroName\"" w487 {
          tunnel: "MacroGroup" -> [_ _ _ _]
          frame "MacroPlay", Default {
          }
          frame "MacroPause" {
          }
          frame "MacroStop" {
          }
          frame "MacroName" {
          }
        }
      }
      event "Go to Next Step": Value Change {
        n248 = event-data() -> ()  [unwired: 1 in, 3 out]
        n249 = call "Table Test Sequencer.vi"("Action"=StateMachineStates_TEST_TDEF."Force Next Step") -> ()  [unwired: 3 in, 8 out]
      }
      event "Go to Previous Step": Value Change {
        n250 = event-data() -> ()  [unwired: 1 in, 3 out]
        n251 = call "Table Test Sequencer.vi"("Action"=StateMachineStates_TEST_TDEF."Force Previous Step") -> ()  [unwired: 3 in, 8 out]
      }
      event "BP Reg Manual": Value Change {
        n252 = event-data() -> ()  [unwired: 1 in, 3 out]
        n253 = Select(t=T17."Enabled" ("Disabled"), s="BP Reg Manual", f=T17."Disabled and Grayed Out" ("Disabled")) -> (s? t:f=w494:T17)
        n254 = property on="BP Regulator" class="Slide (strict)"("DisabledEnum"=w494) -> ()  [unwired: 2 in, 2 out]
      }
      event "Send to Excel": Value Change {
        n255 = event-data() -> ()  [unwired: 1 in, 1 out]
        n256 = call "Queue Command Bundle.vi"("Command"="Send to Excel" ("element")) -> ("main window queue datatype"=w499:T10)  [unwired: 10 in]
        n257 = Enqueue Element(queue=w498, element=w499) -> (queue out=w497:refnum<queue>)  [unwired: 2 in, 2 out]
      }
    }
  }
  n258 = call <vilib>:"Clear Errors.vi"("error in (no error)"=w9) -> ("error out"=w8:errorcluster)  [unwired: 5 in, 1 out]
  n259 = call <vilib>:"DAQmx Stop Task.vi"("task/channels in"=w6, "error in"=w8) -> ("task out"=w5:refnum<k21>, "error out"=w7:errorcluster)  [unwired: 12 in]
  n260 = call <vilib>:"DAQmx Clear Task.vi"("task in"=w5, "error in"=w7) -> ()  [unwired: 13 in, 1 out]
  n261 = flat-sequence {
    tunnel: w14 -> [w501]
    tunnel: w15 -> [w504]
    frame #0 {
      n262 = call <vilib>:"Simple Error Handler.vi"("error in (no error)"=w501) -> ()  [unwired: 4 in, 5 out]
    }
    frame #1 {
      n263 = Wait (ms)(milliseconds to wait=u32 1000) -> ()  [unwired: 1 out]
    }
    frame #2 {
      n264 = call "GLOG_Logger_Methods.vi"("Logger Method"=T19."SHUTDOWN") -> ()  [unwired: 9 in, 2 out]
    }
    frame #3 {
      n265 = Release Queue(queue=w504) -> ()  [unwired: 2 in, 3 out]
    }
    frame #4 {
      n266 = disable-structure shown="RUN_TIME_ENGINE==True" {
        frame condition #0 {
          n267 = Quit LabVIEW() -> ()  [unwired: 1 in]
        }
        frame condition #1 (active) {
          (unwired) TRUE
        }
      }
    }
  }
  "Version" <- "Version 3.0.1\n03/7/2024" ("Version")
